vi "20T_Split_Cluster.vi"(0 "20 T Cluster":T3={"Clamp"=FALSE, "Switch Heater"=FALSE, "Go to Zero"=FALSE, "Go to set"=FALSE, "Go to Hold"=FALSE, "Clamped"=TRUE, "Quenched"=TRUE, "Rate limit"=FALSE, "Persistent"=FALSE, "Hold"=FALSE, "Set"=FALSE, "Zero"=FALSE, "Magnet (T)"=0.0, "Leads (T)"=0.0, "Magnet T (K)"=3.4572, "Switch"=FALSE, "Target (T)"=3.4572, "Setpoint (T)"=3.4572, "Rate (T/min)"=0.0, "Switch Heater 2"=FALSE, "Set Rate"=FALSE} {"Rate (T/min)" format="%6_5f"; "Setpoint (T)" format="%6_5f"; "Target (T)" format="%#4_5f"; "Magnet T (K)" format="%#4_5f"; "Leads (T)" format="%6_5f"}) -> (1 "20 T Statusl":T2={"Clamped"=FALSE, "Quenched"=FALSE, "Rate limit"=FALSE, "Persistent"=FALSE, "Hold"=FALSE, "Set"=FALSE, "Zero"=FALSE, "Magnet (T)"=0.0, "Leads (T)"=0.0, "Magnet T (K)"=3.4572, "Switch"=FALSE} {"Magnet T (K)" format="%#4_5f"; "Leads (T)" format="%6_5f"}, 2 "20 T Control":T1={"Clamp"=FALSE, "Switch Heater"=FALSE, "Go to Zero"=FALSE, "Go to Set"=FALSE, "Go to Hold"=FALSE, "Setpoint (T)"=3.4572, "Rate (T/min)"=0.0, "Set Rate"=FALSE} {"Rate (T/min)" format="%6_5f"; "Setpoint (T)" format="%#4_5f"})   [LabVIEW 2016]
uses:
  Gustav/20T_Cluster.ctl
  Gustav/20T_Status.ctl
  Gustav/20T_Control.ctl
panel:
  # "20 T"
  # "20 T"
  # "20 T"
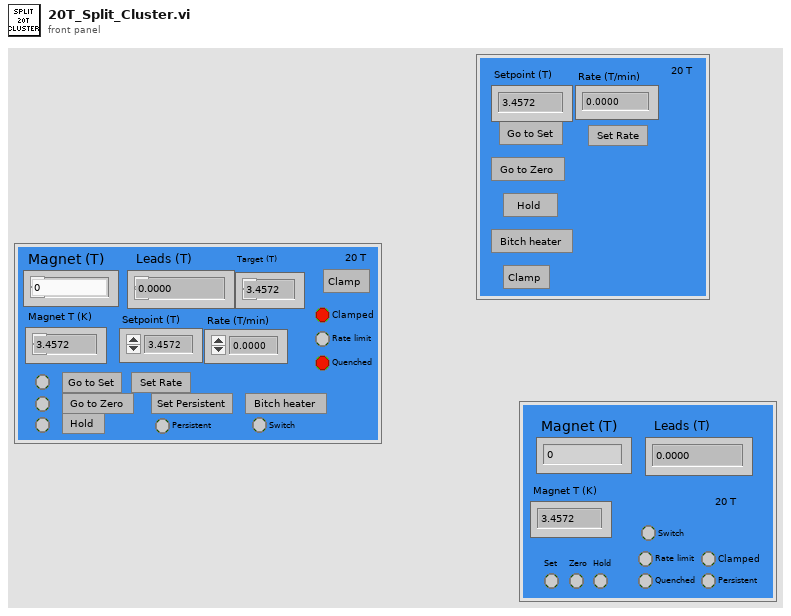
[diagram p1: front panel]
types:
  T1 = typedef "20T_Control.ctl" = cluster{"Clamp":bool, "Switch Heater":bool, "Go to Zero":bool, "Go to Set":bool, "Go to Hold":bool, "Setpoint (T)":dbl, "Rate (T/min)":dbl, "Set Rate":bool}
  T2 = typedef "20T_Status.ctl" = cluster{"Clamped":bool, "Quenched":bool, "Rate limit":bool, "Persistent":bool, "Hold":bool, "Set":bool, "Zero":bool, "Magnet (T)":dbl, "Leads (T)":dbl, "Magnet T (K)":dbl, "Switch":bool}
  T3 = typedef "20T_Cluster.ctl" = cluster{"Clamp":bool, "Switch Heater":bool, "Go to Zero":bool, "Go to set":bool, "Go to Hold":bool, "Clamped":bool, "Quenched":bool, "Rate limit":bool, "Persistent":bool, "Hold":bool, "Set":bool, "Zero":bool, "Magnet (T)":dbl, "Leads (T)":dbl, "Magnet T (K)":dbl, "Switch":bool, "Target (T)":dbl, "Setpoint (T)":dbl, "Rate (T/min)":dbl, "Switch Heater 2":bool, "Set Rate":bool}
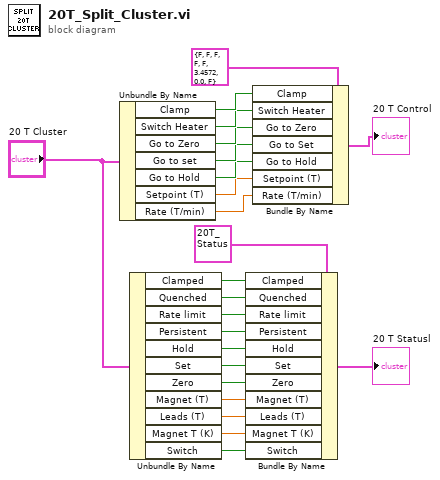
[diagram p0: block diagram]
diagram:
  n1 = Unbundle By Name("20 T Cluster") -> ("Clamp"=w7:bool, "Switch Heater"=w6:bool, "Go to Zero"=w5:bool, "Go to set"=w4:bool, "Go to Hold"=w3:bool, "Setpoint (T)"=w2:dbl, "Rate (T/min)"=w1:dbl)
  n2 = Unbundle By Name("20 T Cluster") -> ("Clamped"=w18:bool, "Quenched"=w17:bool, "Rate limit"=w16:bool, "Persistent"=w15:bool, "Hold"=w14:bool, "Set"=w13:bool, "Zero"=w12:bool, "Magnet (T)"=w11:dbl, "Leads (T)"=w10:dbl, "Magnet T (K)"=w9:dbl, "Switch"=w8:bool)
  n3 = Bundle By Name(cluster=T2 {"Clamped"=FALSE, "Quenched"=FALSE, "Rate limit"=FALSE, "Persistent"=FALSE, "Hold"=FALSE, "Set"=FALSE, "Zero"=FALSE, "Magnet (T)"=0.0, "Leads (T)"=0.0, "Magnet T (K)"=3.4572, "Switch"=FALSE} ("20 T Magnet control"), "Clamped"=w18, "Quenched"=w17, "Rate limit"=w16, "Persistent"=w15, "Hold"=w14, "Set"=w13, "Zero"=w12, "Magnet (T)"=w11, "Leads (T)"=w10, "Magnet T (K)"=w9, "Switch"=w8) -> (→"20 T Statusl":T2)
  n4 = Bundle By Name(cluster=T1 {"Clamp"=FALSE, "Switch Heater"=FALSE, "Go to Zero"=FALSE, "Go to Set"=FALSE, "Go to Hold"=FALSE, "Setpoint (T)"=3.4572, "Rate (T/min)"=0.0, "Set Rate"=FALSE} ("20 T Magnet control"), "Clamp"=w7, "Switch Heater"=w6, "Go to Zero"=w5, "Go to Set"=w4, "Go to Hold"=w3, "Setpoint (T)"=w2, "Rate (T/min)"=w1) -> (→"20 T Control":T1)
